vi "Test SenseHat.Joystick.vi"() -> ()   [LabVIEW 2020]
uses:
  src/RPI.SenseHat.Joystick/TypeDefs/Joystick.ctl
  <vilib>/MakerHub/LINX/Public/Utilities/Open Local.vi
  <vilib>/MakerHub/LINX/LMH-LINX.lvlib
  src/RPI.SenseHat.Joystick/Classes/senseHatJoystick/RPI.SenseHat.Joystick.lvclass
  src/RPI.SenseHat.Joystick/RPI.SenseHat.Joystick.lvlib
panel:
  out "Joystick":T1
  out "Device Name":string
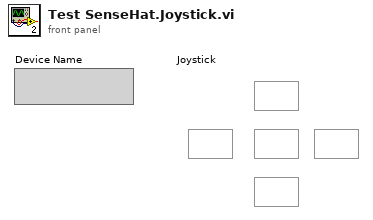
[diagram p1: front panel]
types:
  T1 = typedef "RPI.SenseHat.Joystick.lvlib/Joystick.ctl" = cluster{"Enter":bool, "Down":bool, "Up":bool, "Right":bool, "Left":bool}
  T2 = typedef "LMH-LINX.lvlib/LINX Ref.ctl" = cluster{"IO":T3, "Interface":T4, "LINX Device Config":T5}
  T3 = typedef "LMH-LINX.lvlib/Platform.ctl" = enum16{"Remote", "Local"}
  T4 = typedef "LMH-LINX.lvlib/Interface.ctl" = enum16{"Serial", "TCP"}
  T5 = typedef "LMH-LINX.lvlib/Device.lvlib/LINX Device Config.ctl" = cluster{"Interface":T4, "COM Port":refnum<visa-resource-name>, "TCP Configuration":T6, "Device Family":u8, "Device ID":u8, "Device Name":string, "TCP Ref":refnum<k5>, "Channels":T7}
  T6 = typedef "LMH-LINX.lvlib/Device.lvlib/TCP Config.ctl" = cluster{"IP Address":string, "Port":u16}
  T7 = typedef "LMH-LINX.lvlib/Channels.ctl" = cluster{"DI":u8[], "DO":u8[], "AI":u8[], "AO":u8[], "PWM":u8[], "QE":u8[], "UART":u8[], "I2C 2":u8[], "SPI":u8[], "CAN":u8[], "Servo":u8[], "AI Ref (V)":dbl, "AI Resolution (Bits)":u8, "AO Ref (V)":dbl, "AO Resolution (Bits)":u8}
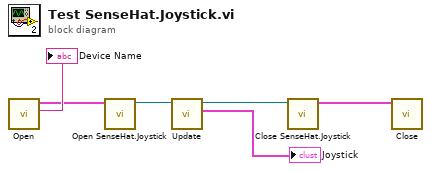
[diagram p0: block diagram]
diagram:
  n1 = call-poly <vilib>:"Open.vi"() -> ("Device Name"=→"Device Name":string, "LINX Resource"=w5:T2)  [unwired: 9 in, 1 out]
  n2 = call "Open SenseHat.Joystick.vi"("LINX Resource"=w5) -> ("senseHatJoystick out"=w3:refnum<class "RPI.SenseHat.Joystick.lvclass">)  [unwired: 9 in, 1 out]
  n3 = call "Update.vi"("senseHatJoystick in"=w3) -> ("Joystick"=→"Joystick":T1, "senseHatJoystick out"=w2:refnum<class "RPI.SenseHat.Joystick.lvclass">)  [unwired: 8 in, 1 out]
  n4 = call "Close SenseHat.Joystick.vi"("senseHatJoystick in"=w2) -> ("LINX Resource"=w4:T2)  [unwired: 9 in, 1 out]
  n5 = call <vilib>:"Close.vi"("LINX Resource"=w4) -> ()  [unwired: 10 in, 1 out]
